vi "ResizeIfNeeded.vi"(1 "Size":i32[](array[numeric]), 2 "Table":string[][](array[string])) -> (0 "Table out":string[][](array[string]))   [LabVIEW 2012]
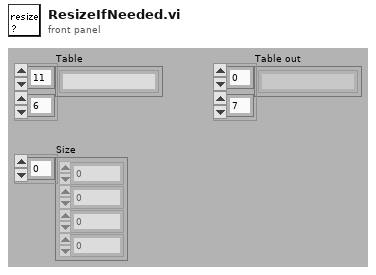
[diagram p1: front panel]
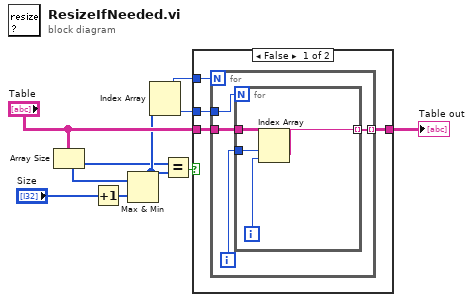
[diagram p0: block diagram]
diagram:
  n1 = Array Size(array="Table") -> (size(s)=w2:i32[])
  n2 = Increment(x="Size") -> (x+1=w8:i32[])
  n3 = Max & Min(x=w2, y=w8) -> (max(x,y)=w5:i32[])  [unwired: 1 out]
  n4 = Index Array(array=w5) -> (element #1=w6:i32, element #2=w7:i32)  [unwired: 2 in]
  n5 = Equal?(x=w2, y=w5) -> (x = y?=w3:bool)
  n6 = case shown="False" w3 {
    tunnel: [w10 w22] -> w4
    tunnel: "Table" -> [w11 w22]
    tunnel: w6 -> [w13 _]
    tunnel: w7 -> [w12 _]
    frame False {
      n7 = for {
        N: w13 -> [_]
        tunnel: w12 -> [w17]
        tunnel: w11 -> [w16]
        tunnel: [w14] -> w10 mode=indexing
        i -> [w15]
        n8 = for {
          N: w17 -> [_]
          tunnel: w16 -> [w21]
          tunnel: w15 -> [w20]
          tunnel: [w18] -> w14 mode=indexing
          i -> [w19]
          n9 = Index Array(array=w21, index (row)=w20, index (col)=w19) -> (element=w18:string)
        }
      }
    }
    frame True {
    }
  }
  "Table out" <- w4
